vi "Battery charger.vi"() -> ()   [LabVIEW 2018]
panel:
  out "String":string
  out "Boolean":bool
  out "Slide":u8(slide) scale=0.0..100.0
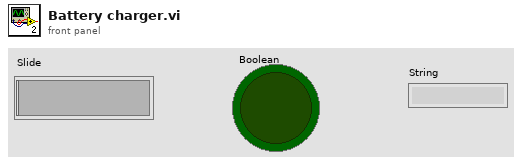
[diagram p1: front panel]
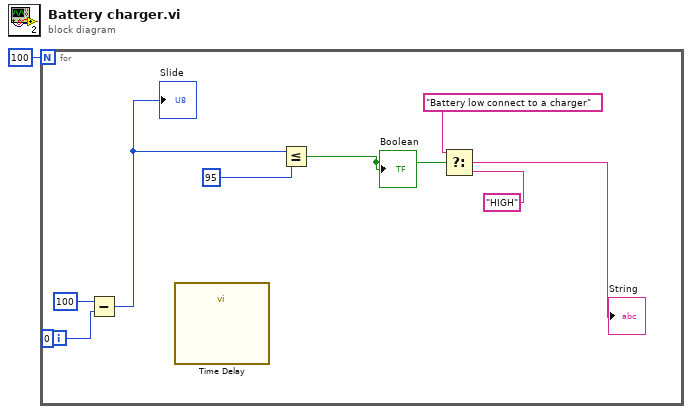
[diagram p0: block diagram]
diagram:
  n1 = for {
    N: 100 -> [_]
    i -> [w8]
    (unwired) 0
    n2 = Subtract(x=100, y=w8) -> (x-y=w6:i32)
    "Slide" <- w6
    n3 = call "Time Delay"() -> ()  [unwired: 11 in, 1 out]
    n4 = Less Or Equal?(x=w6, y=95) -> (x <= y?=w5:bool)
    "Boolean" <- w5
    n5 = Select(t="Battery low connect to a charger", s=w5, f="HIGH") -> (s? t:f=→"String":string)
  }
